vi "D_Window_Settings.vi"(7 "Window Number (0...15)":i32, 8 "error in (no error)":errorcluster, 9 "YPixelShift":i32, 10 "XPixelShift":i32, 11 "Monitor mumber":i32=1) -> (0 "error out":errorcluster)   [LabVIEW 2016]
uses:
  SLM_Control_VI_source/Image_Control.dll
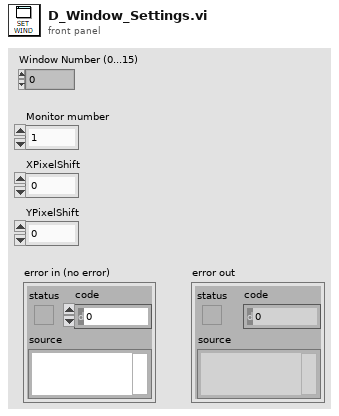
[diagram p1: front panel]
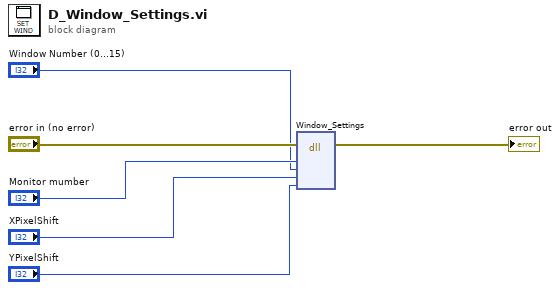
[diagram p0: block diagram]
diagram:
  n1 = dll-call lib="C:/Users/hs5921/Desktop/SLM_Control_VI_source/Image_Control.dll" fn="Window_Settings"(error in="error in (no error)", "Monitor_Number"="Monitor mumber", "Window_Number_0_to_15"="Window Number (0...15)", "XPixelShift"="XPixelShift", "YPixelShift"="YPixelShift") -> (error out=→"error out":errorcluster)  [unwired: 7 in, 1 out]
